vi "control_stepsize.vi"(4 "#Iterations":refnum<vi>, 6 "Stepsize":refnum<vi>, 9 "Endtime":dbl, 11 "Starttime":dbl) -> ()   [LabVIEW 2019]
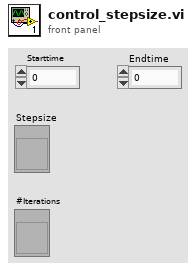
[diagram p1: front panel]
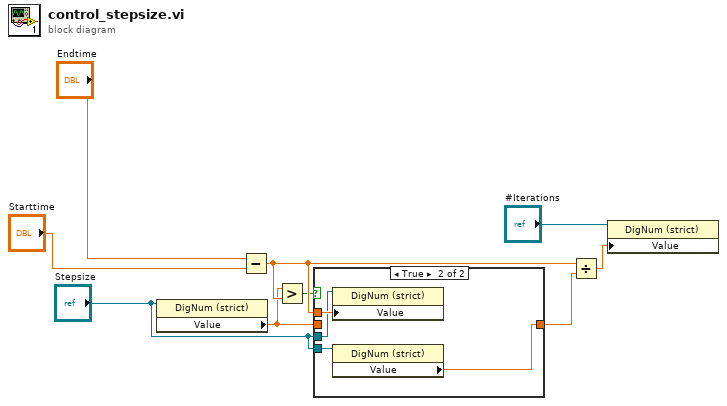
[diagram p0: block diagram]
diagram:
  n1 = property on="Property Node" class="DigNum (strict)"(reference="Stepsize") -> ("Value"=w7:dbl)  [unwired: 1 in, 2 out]
  n2 = Subtract(x="Endtime", y="Starttime") -> (x-y=w9:dbl)
  n3 = Greater?(x=w7, y=w9) -> (0:w5:bool)
  n4 = case shown="True" w5 {
    tunnel: w9 -> [_ w14]
    tunnel: [w10 w13] -> w8
    tunnel: w7 -> [w10 _]
    tunnel: "Stepsize" -> [_ w12]
    tunnel: "Stepsize" -> [_ w11]
    frame False {
    }
    frame True {
      n5 = property on="Property Node" class="DigNum (strict)"(reference=w12, "Value"=w14) -> ()  [unwired: 1 in, 2 out]
      n6 = property on="Property Node" class="DigNum (strict)"(reference=w11) -> ("Value"=w13:dbl)  [unwired: 1 in, 2 out]
    }
  }
  n7 = Divide(x=w9, y=w8) -> (x/y=w6:dbl)
  n8 = property on="Property Node" class="DigNum (strict)"(reference="#Iterations", "Value"=w6) -> ()  [unwired: 1 in, 2 out]
